vi "PVCamPropertyChangedCallbackForHistogram.vi"(4 "?":refnum<vi>, 5 "Event Data":cluster{"sender":refnum<k24>, "e":refnum<k24>}, 6 "Control Ref":refnum<k24>, 7 "Event Common Data":T1) -> ()   [LabVIEW 2018]
uses:
  D:/SVN/PM/sdk/AppSamples/LabVIEWSamples/trunk/Release/2018/Dependencies/PVCamNET.dll
  Dependencies/PVCamNET.dll
  PVCamGlobalVariables.vi
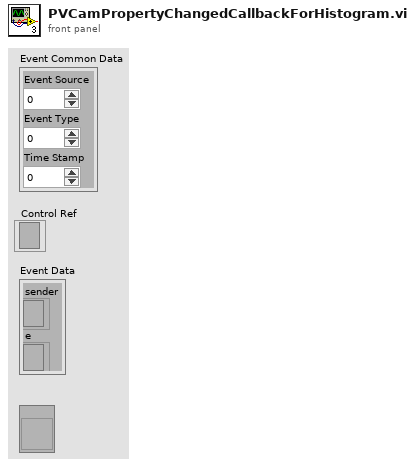
[diagram p1: front panel]
types:
  T1 = cluster{"Event Source":i32, "Event Type":u32, "Time Stamp":u32}
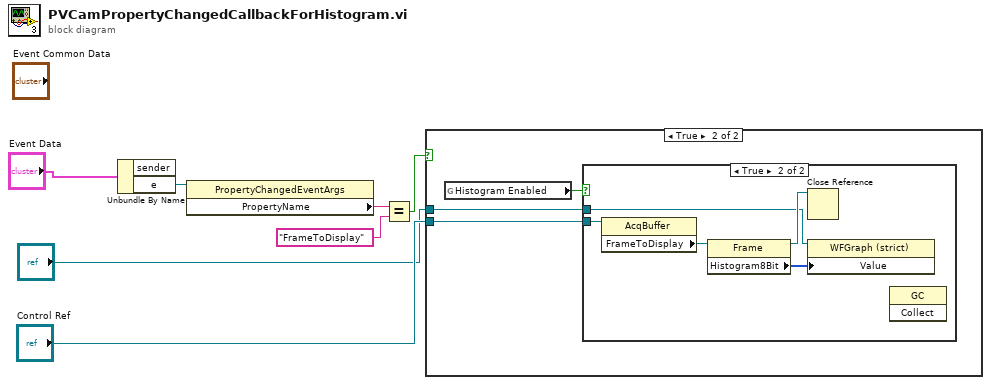
[diagram p0: block diagram]
diagram:
  n1 = Unbundle By Name("Event Data") -> ("e"=w7:refnum<k24>)  [unwired: 1 out]
  n2 = property class="PropertyChangedEventArgs"(reference=w7) -> ("PropertyName"=w6:string)  [unwired: 1 in, 2 out]
  n3 = Equal?(x=w6, y="FrameToDisplay") -> (x = y?=w3:bool)
  n4 = case shown="True" w3 {
    tunnel: "Control Ref" -> [_ w10]
    tunnel: "?" -> [_ w9]
    frame False {
    }
    frame True {
      n5 = global read "PVCamGlobalVariables.vi" "Histogram Enabled"() -> (w8:bool)
      n6 = case shown="True" w8 {
        tunnel: w10 -> [_ w15]
        tunnel: w9 -> [_ w12]
        frame False {
        }
        frame True {
          n7 = property class="AcqBuffer"(reference=w15) -> ("FrameToDisplay"=w14:refnum<k24>)  [unwired: 1 in, 2 out]
          n8 = property class="Frame"(reference=w14) -> (reference out=w13:refnum<k24>, "Histogram8Bit"=w11:u32[])  [unwired: 1 in, 1 out]
          n9 = Close Reference(reference=w13) -> ()  [unwired: 1 in, 1 out]
          n10 = property class="WFGraph (strict)"(reference=w12, "Value"=w11) -> ()  [unwired: 1 in, 2 out]
          n11 = invoke class="GC" method="Collect"() -> ()  [unwired: 3 in, 3 out]
        }
      }
    }
  }
